vi "Tetra_Read Imon.vi"(0 "COMPORT":refnum<visa-resource-name>="COM4", 1 "ini limits directory (if blank will skip)":path=path "C:/RageATE-Tetra/Support", 4 "rev_c(t)":bool=TRUE, 5 "error in (no error)":errorcluster={"status"=FALSE, "code"=1073676418, "source"="VISA Close in Tetra_TX-ATTEN_Setup.vi"}, 7 "Open Ser(t)":bool, 9 "Meas_Limits":bool, 11 "Clear errors in(t)":bool=TRUE, 13 "Close Ser(t)":bool) -> (6 "rdiv(i)":dbl[](array[numeric])=[0.496, 0.124, 0.318, 0.209, 1.171, 1.122], 10 "rdiv(v)":dbl[](array[numeric])=[3.456, 5.48, 2.896, 2.928, 2.344, 1.448], 12 "Result  0|1[PASS/FAIL]: dcv(7b) dci(7b)":string="1  -1", 14 "comport":refnum<visa-resource-name>="COM4", 15 "Fail?(t)":bool, 19 "error out":errorcluster)   [LabVIEW 2018]
panel:
  out "Timeout":bool caption="Time has Elapsed"
  in  "Tab Control":T1(tab)
  in  "rdiv(v)_lim":dbl[][](array[numeric])
  in  "rdiv(i)_lim":dbl[][](array[numeric])
  out "sw_dcv_good":bool[](array[boolean])
  out "sw_dci_good":bool[](array[boolean])
  out "Names":string[](array[string])=["sw3p6", "sw5p5", "sw2p8a", "sw2p8b", "sw2p4", "sw1p4"]
  out "concatenated string 2":string="rdiv\r\n0)  sw3p6:   496 mA  3456 mV\r\n1)  sw5p5:   124 mA  5480 mV\r\n2) sw2p8a:   318 mA  2896 mV\r\n3) sw2p8b:   209 mA  2928 mV\r\n4)  sw2p4:  1171 mA  2344 mV\r\n5)  sw1p4:  1122 mA  1448 mV\r\n>"
  # "This vi will query the on board i2c current monitors on Tetra WAM rev B0.5 via FPGA"
  # "Readback"
  # "Set Limits"
  # "LSL"
  # "HSL"
  # "LSL"
  # "HSL"
  # "5083549_Release_B_05.PDF"
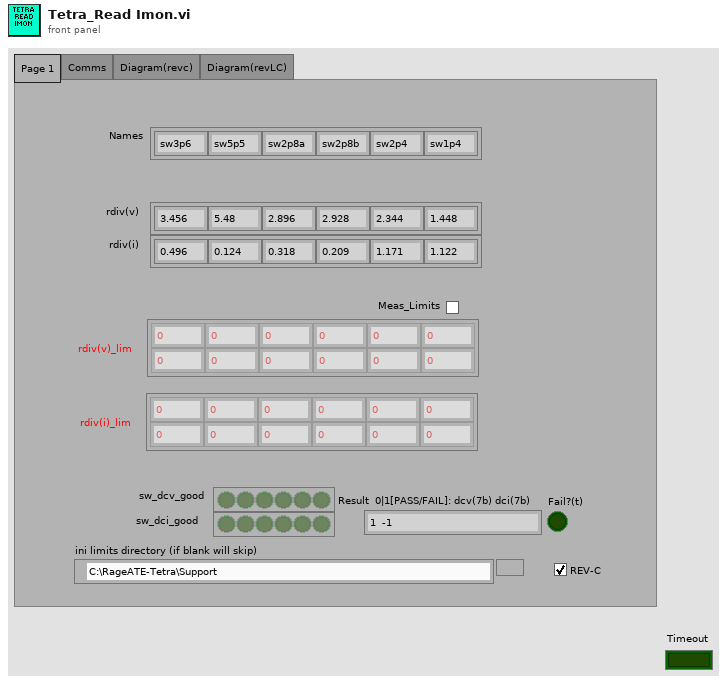
[diagram p1: front panel]
types:
  T1 = enum32{"Page 1", "Comms", "Diagram(revc)", "Diagram(revLC)"}
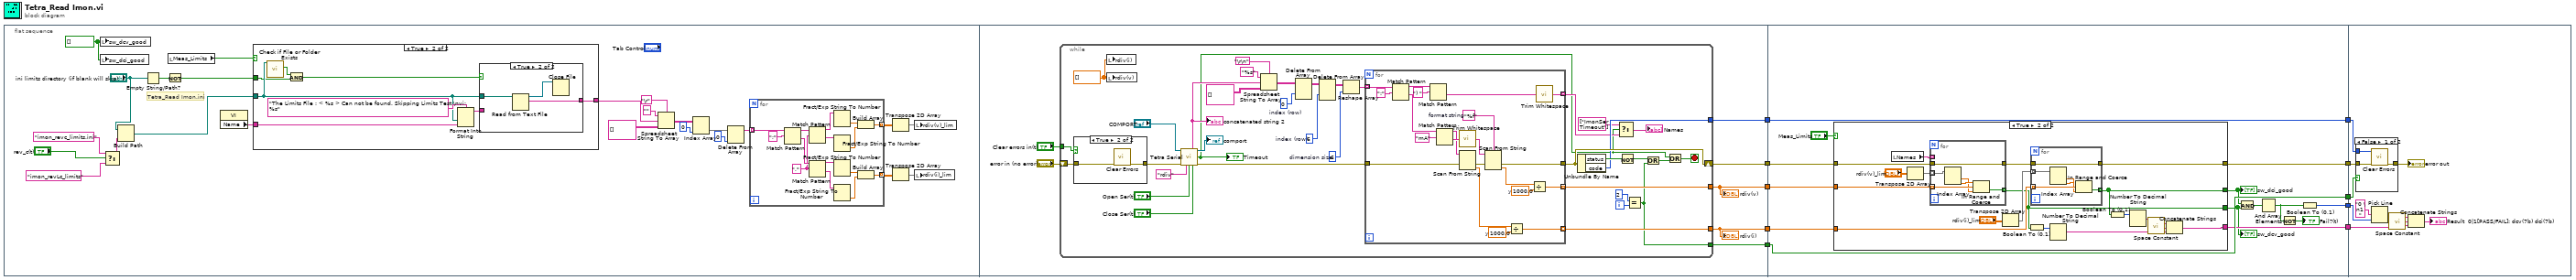
[diagram p0: block diagram]
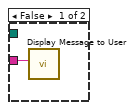
[diagram p3: hidden frame]
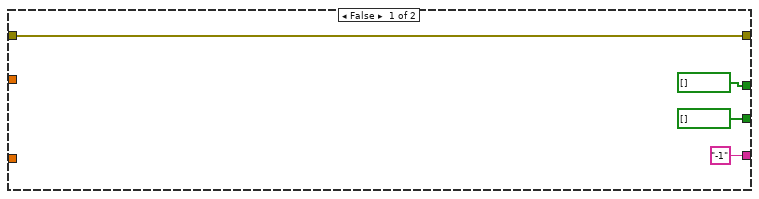
[diagram p5: hidden frame]
diagram:
  n1 = flat-sequence {
    tunnel: [w66] -> w10
    tunnel: [w65] -> w9
    tunnel: [w64] -> w8
    tunnel: [w63] -> w7
    tunnel: [w62] -> w6
    tunnel: w10 -> [w142]
    tunnel: w9 -> [w138]
    tunnel: w8 -> [w141]
    tunnel: w7 -> [w140]
    tunnel: w6 -> [w139]
    tunnel: [w142] -> w5
    tunnel: [w137] -> w4
    tunnel: [w141] -> w3
    tunnel: [w136] -> w2
    tunnel: [w132] -> w1
    tunnel: w5 -> [w185]
    tunnel: w4 -> [w184]
    tunnel: w3 -> [w183]
    tunnel: w2 -> [w182]
    tunnel: w1 -> [w178]
    frame #0 {
      w34 = bool[] [] ("sw_dci_good")
      # "Tetra_Read Imon.ini"
      n2 = local write "sw_dcv_good"(w34) -> ()
      n3 = local write "sw_dci_good"(w34) -> ()
      n4 = Select(t="imon_revc_limits.ini" ("name or relative path"), s="rev_c(t)", f="imon_revLc_limits" ("name or relative path")) -> (s? t:f=w13:string)
      n5 = Build Path(base path="ini limits directory (if blank will skip)", name or relative path=w13) -> (appended path=w15:path)
      n6 = Empty String/Path?(string/path="ini limits directory (if blank will skip)") -> (empty?=w32:bool)
      n7 = Not(x=w32) -> (.not. x?=w30:bool)
      n8 = local read "Meas_Limits"() -> (w31:bool)
      n9 = property class="VI"() -> ("Name"=w33:string)  [unwired: 2 in, 2 out]
      n10 = case shown="True" w31 {
        tunnel: w15 -> [_ w54]
        tunnel: w33 -> [_ w53]
        tunnel: w30 -> [_ w51]
        tunnel: [_ w50] -> w29
        frame False {
        }
        frame True {
          n11 = call <vilib>:"Check if File or Folder Exists.vi"("path"=w54) -> ("file or folder exists?"=w57:bool)  [unwired: 8 in, 2 out]
          n12 = And(x=w57, y=w51) -> (x .and. y?=w52:bool)
          n13 = Format Into String(format string="The Limits File : < %s > Can not be found. Skipping Limits Test \nvi: %s", w54, w53) -> (resulting string=w55:string)  [unwired: 2 in, 1 out]
          n14 = case shown="True" w52 {
            tunnel: w54 -> [_ w61]
            tunnel: w55 -> [w58 _]
            tunnel: [_ w60] -> w50
            frame False {
              n15 = call "Display Message to User"("Message"=w58) -> ()  [unwired: 9 in, 2 out]
            }
            frame True {
              n16 = Read from Text File(file (use dialog)=w61) -> (refnum out=w59:refnum<file>, text=w60:string)  [unwired: 3 in, 2 out]
              n17 = Close File(refnum=w59) -> ()  [unwired: 1 in, 2 out]
            }
          }
        }
      }
      n18 = Spreadsheet String To Array(delimiter (Tab)="\r", format string="", spreadsheet string=w29, array type (2D Dbl)=string[][] []) -> (array=w25:string[][])
      n19 = Index Array(array=w25, index (col)=0 ("disabled index (col)")) -> (element=w24:string[])  [unwired: 1 in]
      n20 = Delete From Array(array=w24, index=0) -> (array with subset deleted=w22:string[])  [unwired: 1 in, 1 out]
      n21 = for {
        tunnel: w22 -> [w49] mode=indexing
        tunnel: [w36] -> w19 mode=indexing
        tunnel: [w35] -> w20 mode=indexing
        w45 = "," ("regular expression")
        n22 = Match Pattern(string=w49, regular expression=";") -> (before substring=w47:string, after substring=w46:string)  [unwired: 1 in, 2 out]
        n23 = Match Pattern(string=w47, regular expression=w45) -> (before substring=w44:string, after substring=w43:string)  [unwired: 1 in, 2 out]
        n24 = Match Pattern(string=w46, regular expression=w45) -> (before substring=w42:string, after substring=w41:string)  [unwired: 1 in, 2 out]
        n25 = Fract/Exp String To Number(string=w44) -> (number=w40:dbl)  [unwired: 3 in, 1 out]
        n26 = Fract/Exp String To Number(string=w43) -> (number=w39:dbl)  [unwired: 3 in, 1 out]
        n27 = Fract/Exp String To Number(string=w42) -> (number=w38:dbl)  [unwired: 3 in, 1 out]
        n28 = Fract/Exp String To Number(string=w41) -> (number=w37:dbl)  [unwired: 3 in, 1 out]
        n29 = Build Array(w40, w39) -> (w36:dbl[])
        n30 = Build Array(w38, w37) -> (w35:dbl[])
      }
      n31 = Transpose 2D Array(2D array=w19) -> (transposed array=w18:dbl[][])
      n32 = Transpose 2D Array(2D array=w20) -> (transposed array=w17:dbl[][])
      n33 = local write "rdiv(v)_lim"(w18) -> ()
      n34 = local write "rdiv(i)_lim"(w17) -> ()
    }
    frame #1 {
      n35 = while {
        tunnel: [w104] -> w62
        tunnel: [w103] -> w63
        tunnel: "Clear errors in(t)" -> [w100]
        shift-right: [w82] -> w65
        shift-left: "error in (no error)" -> [w101]
        tunnel: [w77] -> w66
        tunnel: [w76] -> w64
        i -> [w80]
        stop <- w73 stop-if-true
        w88 = 6  # dimension size
        w90 = 6  # index (row)
        w92 = 0  # index (row)
        w98 = dbl[] []
        n36 = case shown="True" w100 {
          tunnel: [w126 w128] -> w99
          tunnel: w101 -> [w126 w127]
          frame False {
          }
          frame True {
            n37 = call <vilib>:"Clear Errors.vi"("error in (no error)"=w127) -> ("error out"=w128:errorcluster)  [unwired: 5 in, 1 out]
          }
        }
        n38 = local write "rdiv(i)"(w98) -> ()
        n39 = local write "rdiv(v)"(w98) -> ()
        n40 = call "Tetra Serial.vi"("COMPORT"="COMPORT", "error in (no error)"=w99, "Command"="rdiv", "Open Ser(t)"="Open Ser(t)", "Close Ser(t)"="Close Ser(t)") -> ("output"=w85:string, "comport"=→"comport":refnum<visa-resource-name>, "Timeout"=w69:bool, "error out"=w84:errorcluster)  [unwired: 6 in, 1 out]
        "concatenated string 2" <- w85
        "Timeout" <- w69
        n41 = Spreadsheet String To Array(delimiter (Tab)="\r\n", format string="%s", spreadsheet string=w85, array type (2D Dbl)=string[][] []) -> (array=w93:string[][])
        n42 = Delete From Array(array=w93, index (row)=w92) -> (array with subset deleted=w91:string[][])  [unwired: 2 in, 1 out]
        n43 = Delete From Array(array=w91, index (row)=w90) -> (array with subset deleted=w89:string[][])  [unwired: 2 in, 1 out]
        n44 = Reshape Array(w89, w88) -> (w87:string[])
        n45 = for {
          tunnel: w87 -> [w125] mode=indexing
          tunnel: [w116] -> w104 mode=indexing
          tunnel: [w113] -> w103 mode=indexing
          tunnel: [w109] -> w82
          tunnel: w84 -> [w111]
          tunnel: [w105] -> w72 mode=indexing
          w117 = 1000.0  # y
          w119 = 1000.0  # y
          w121 = "%f"  # format string
          n46 = Match Pattern(string=w125, regular expression=":") -> (before substring=w108:string, after substring=w120:string)  [unwired: 1 in, 2 out]
          n47 = Match Pattern(string=w108, regular expression=") ") -> (after substring=w106:string)  [unwired: 1 in, 3 out]
          n48 = Match Pattern(string=w120, regular expression="mA") -> (before substring=w112:string, after substring=w118:string)  [unwired: 1 in, 2 out]
          n49 = call <vilib>:"Trim Whitespace.vi"("string"=w118) -> ("trimmed string"=w115:string)  [unwired: 1 in]
          n50 = Scan From String(input string=w112, error in=w111) -> (error out=w110:errorcluster, output 1=w114:dbl)  [unwired: 3 in, 2 out]
          n51 = Scan From String(format string=w121, input string=w115, error in=w110) -> (error out=w109:errorcluster, output 1=w122:dbl)  [unwired: 2 in, 2 out]
          n52 = Divide(x=w114, y=w117) -> (x/y=w113:dbl)
          n53 = Divide(x=w122, y=w119) -> (x/y=w116:dbl)
          n54 = call <vilib>:"Trim Whitespace.vi"("string"=w106) -> ("trimmed string"=w105:string)  [unwired: 1 in]
        }
        n55 = Unbundle By Name(w82) -> ("status"=w81:bool, "code"=w76:i32)
        n56 = Select(t=string[] ["ImonSer Timeout"], s=w69, f=w72) -> (s? t:f=→"Names":string[])
        n57 = Not(x=w81) -> (.not. x?=w78:bool)
        n58 = Equal?(x=2, y=w80) -> (x = y?=w77:bool)
        n59 = Or(x=w78, y=w77) -> (x .or. y?=w83:bool)
        n60 = Or(x=w69, y=w83) -> (x .or. y?=w73:bool)
      }
      "rdiv(v)" <- w62
      "rdiv(i)" <- w63
    }
    frame #2 {
      n61 = case shown="True" "Meas_Limits" {
        tunnel: w140 -> [_ w162]
        tunnel: w139 -> [_ w161]
        tunnel: w138 -> [w146 w157]
        tunnel: [w146 w155] -> w137
        tunnel: ["-1" w149] -> w136
        tunnel: [bool[] [] w148] -> w134
        tunnel: [bool[] [] w147] -> w133
        frame False {
        }
        frame True {
          n62 = local read "Names"() -> (w158:string[])
          n63 = Transpose 2D Array(2D array="rdiv(v)_lim") -> (transposed array=w164:dbl[][])
          n64 = for {
            tunnel: [w170] -> w147 mode=indexing
            tunnel: w164 -> [w169] mode=indexing
            tunnel: w161 -> [w168] mode=indexing
            tunnel: w158 -> [_] mode=indexing
            tunnel: w157 -> [w165]
            tunnel: [w165] -> w156
            n65 = Index Array(array=w169) -> (element #1=w166:dbl, element #2=w167:dbl)  [unwired: 2 in]
            n66 = In Range and Coerce(upper limit=w167, x=w168, lower limit=w166) -> (In Range?=w170:bool)  [unwired: 1 out]
          }
          n67 = Transpose 2D Array(2D array="rdiv(i)_lim") -> (transposed array=w160:dbl[][])
          n68 = Boolean To (0,1)(Boolean=w147) -> (0, 1=w151:i16[])
          n69 = for {
            tunnel: [w176] -> w148 mode=indexing
            tunnel: w162 -> [w175] mode=indexing
            tunnel: w160 -> [w172] mode=indexing
            tunnel: w156 -> [w171]
            tunnel: [w171] -> w155
            n70 = Index Array(array=w172) -> (element #1=w174:dbl, element #2=w173:dbl)  [unwired: 2 in]
            n71 = In Range and Coerce(upper limit=w173, x=w175, lower limit=w174) -> (In Range?=w176:bool)  [unwired: 1 out]
          }
          n72 = Number To Decimal String(number=w151) -> (decimal integer string=w153:string[])  [unwired: 1 in]
          n73 = Boolean To (0,1)(Boolean=w148) -> (0, 1=w150:i16[])
          n74 = Number To Decimal String(number=w150) -> (decimal integer string=w152:string[])  [unwired: 1 in]
          n75 = call <vilib>:"Space Constant.vi"() -> ("String"=w154:string)
          n76 = Concatenate Strings(w152, w154, w153) -> (w149:string)
        }
      }
      "sw_dci_good" <- w134
      "sw_dcv_good" <- w133
      n77 = And(x=w134, y=w133) -> (x .and. y?=w131:bool[])
      n78 = And Array Elements(Boolean array=w131) -> (logical AND=w130:bool)
      n79 = Not(x=w130) -> (.not. x?=→"Fail?(t)":bool)
      n80 = Boolean To (0,1)(Boolean=w130) -> (0, 1=w132:i16)
    }
    frame #3 {
      n81 = case shown="False" w185 {
        tunnel: w184 -> [w189 w190]
        tunnel: [w188 w190] -> w186
        tunnel: w183 -> [w187 _]
        frame False {
          n82 = call <vilib>:"Clear Errors.vi"("error in (no error)"=w189, "specific error code to clear (0: all)"=w187) -> ("error out"=w188:errorcluster)  [unwired: 4 in, 1 out]
        }
        frame True {
        }
      }
      "error out" <- w186
      n83 = Pick Line(multi-line string="0 \n1 ", line index=w178) -> (output string=w177:string)  [unwired: 1 in]
      n84 = call <vilib>:"Space Constant.vi"() -> ("String"=w180:string)
      n85 = Concatenate Strings(w177, w180, w182) -> (→"Result  0|1[PASS/FAIL]: dcv(7b) dci(7b)":string)
    }
  }
